vi "get queues.vi"(11 "communicator in":refnum<class "communicator.lvclass">) -> (2 "to this":refnum<class "identifying queue.lvclass">, 3 "to parent":refnum<class "identifying queue.lvclass">)   [LabVIEW 2015, in "communicator.lvclass"]
uses:
  communicator.lvclass
  communicator queue/identifying queue.lvclass
  communicator.lvclass/communicator.ctl
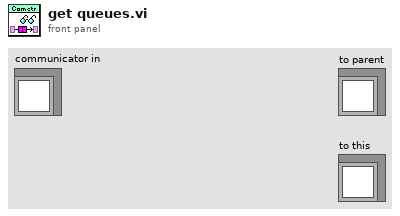
[diagram p1: front panel]
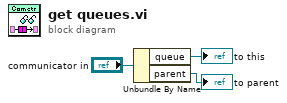
[diagram p0: block diagram]
diagram:
  n1 = Unbundle By Name("communicator in") -> ("queue"=→"to this":refnum<class "identifying queue.lvclass">, "parent"=→"to parent":refnum<class "identifying queue.lvclass">)
